vi "Open Controller matrix.vi"(1 "file path (dialog if empty)":path) -> (0 "Cluster":T1)   [LabVIEW 2018]
uses:
  controls/Controller.ctl
  Real-Time/Control Algorithm/Control Algorithm Selection.ctl
  <vilib>/Utility/file.llb/Read Delimited Spreadsheet (DBL).vi
panel:
  out "all rows":dbl[][](array[numeric]) format="%#_24g"
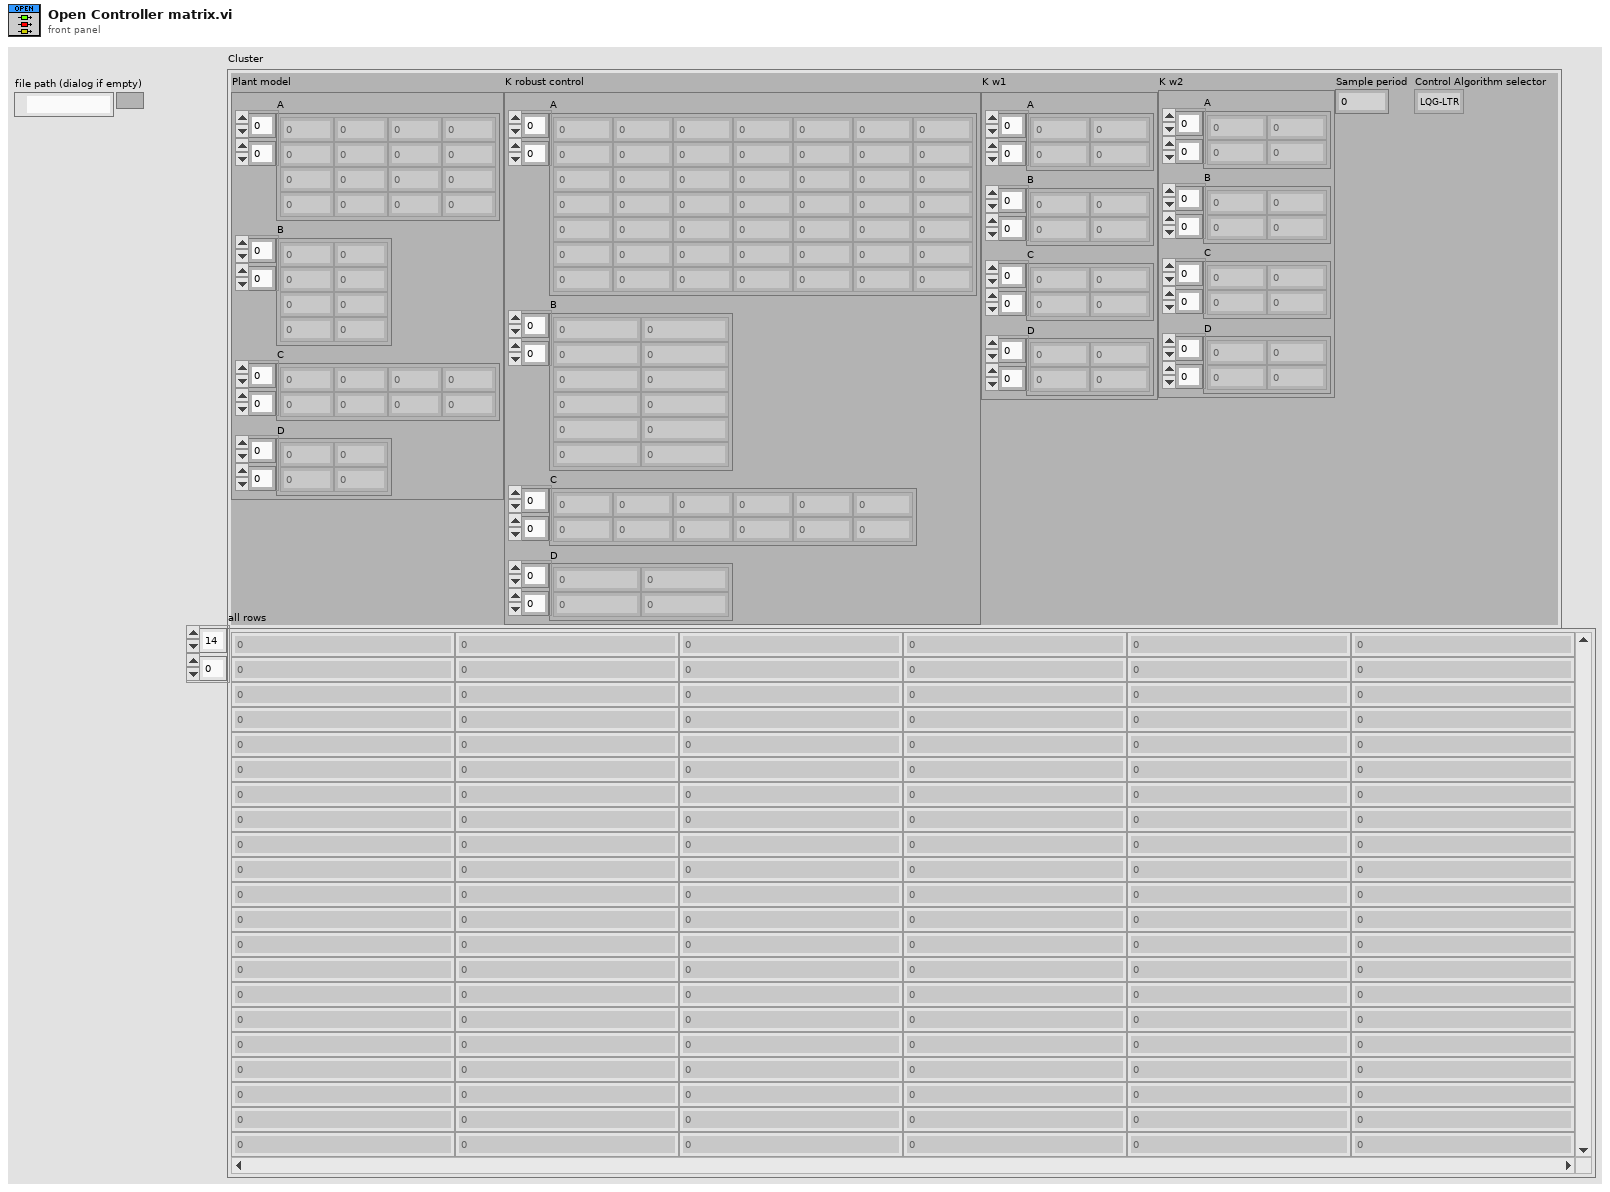
[diagram p1: front panel]
types:
  T1 = typedef "Controller.ctl" = cluster{"Plant model":cluster{"A":dbl[][], "B":dbl[][], "C":dbl[][], "D":dbl[][]}, "K robust control":cluster{"A":dbl[][], "B":dbl[][], "C":dbl[][], "D":dbl[][]}, "K w1":cluster{"A":dbl[][], "B":dbl[][], "C":dbl[][], "D":dbl[][]}, "K w2":cluster{"A":dbl[][], "B":dbl[][], "C":dbl[][], "D":dbl[][]}, "Sample period":dbl, "Control Algorithm selector":T2}
  T2 = typedef "Control Algorithm Selection.ctl" = enum16{"LQG-LTR", "Hinf"}
  T3 = cluster{"A":dbl[][], "B":dbl[][], "C":dbl[][], "D":dbl[][]}
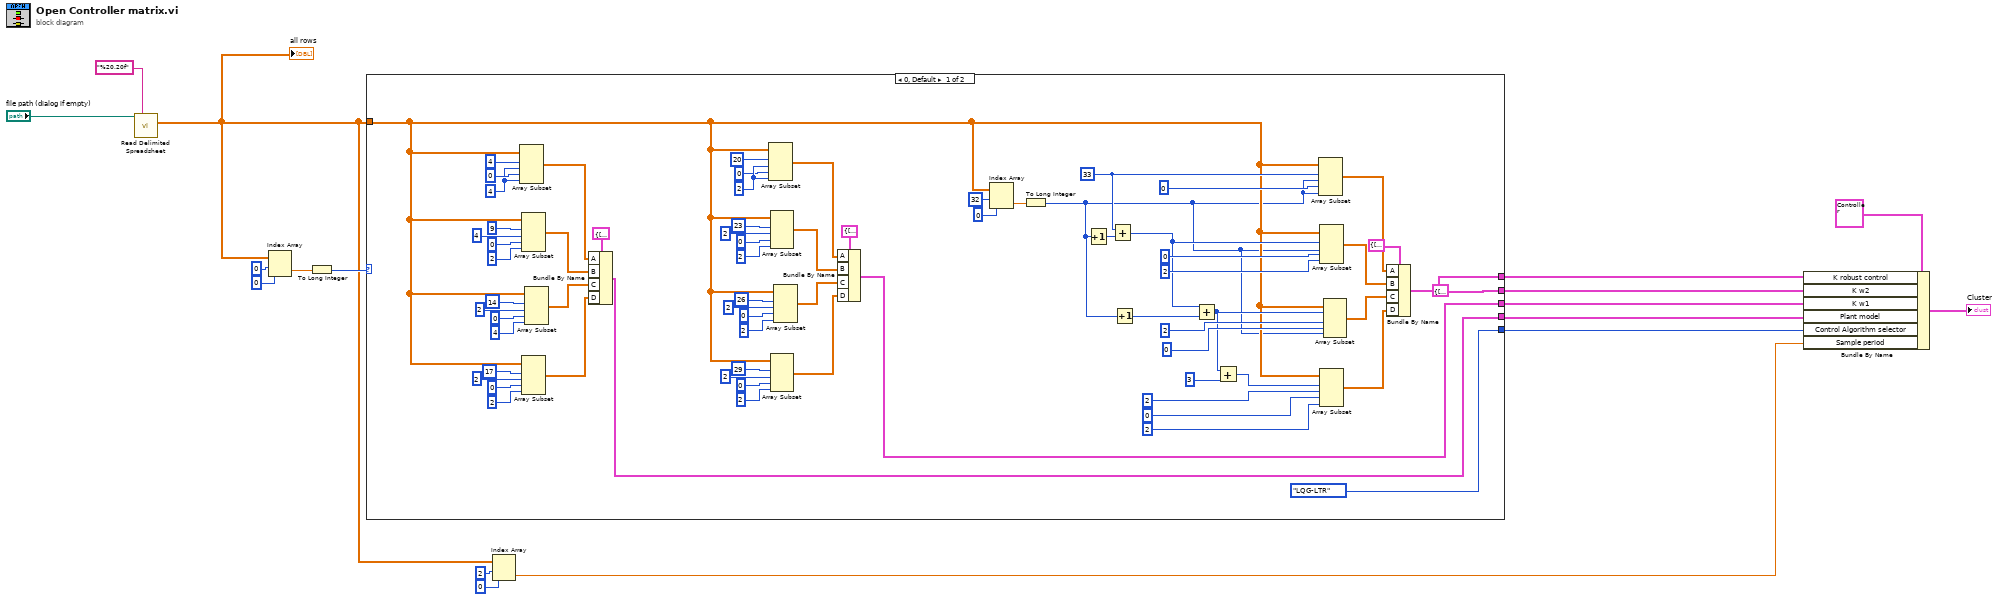
[diagram p0: block diagram]
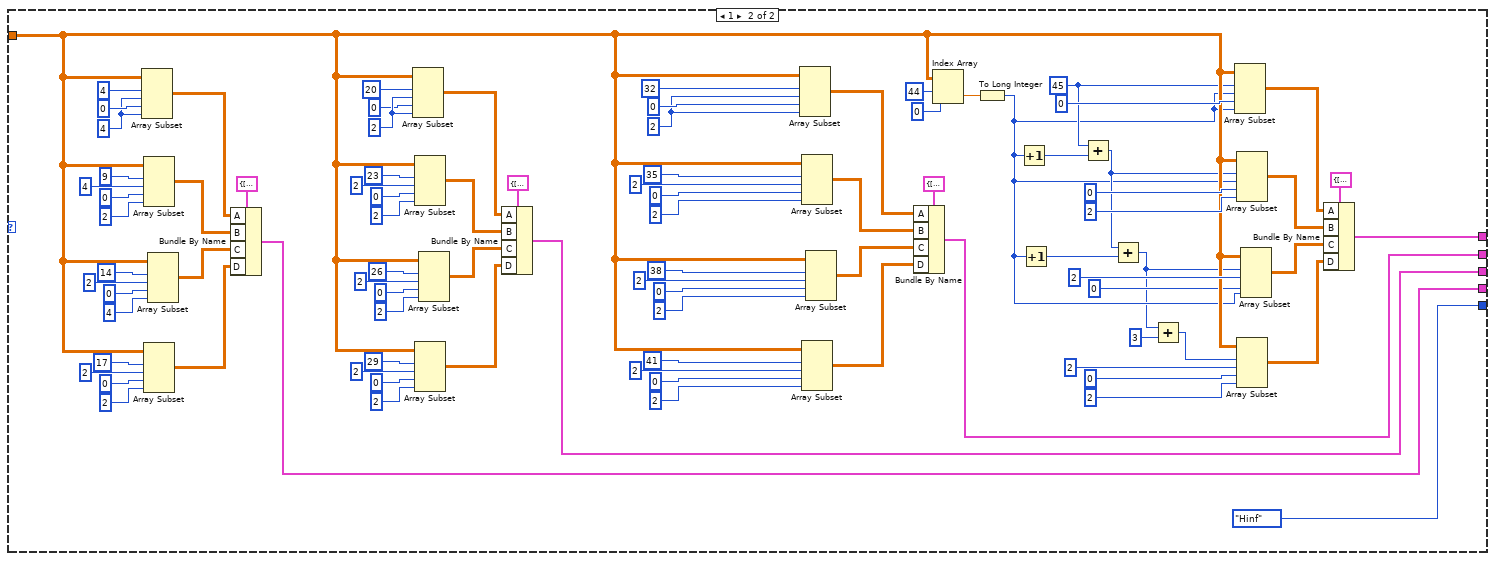
[diagram p2: hidden frame]
diagram:
  n1 = call-poly <vilib>:"Read Delimited Spreadsheet.vi"("file path (dialog if empty)"="file path (dialog if empty)", "format (%.3f)"="%20.20f") -> ("all rows"=w10:dbl[][])  [unwired: 8 in, 5 out]
  "all rows" <- w10
  n2 = Index Array(array=w10, index (row)=0, index (col)=0 ("disabled index (col)")) -> (element=w12:dbl)
  n3 = To Long Integer(number=w12) -> (32bit integer=w11:i32)
  n4 = case shown="0, Default" w11 {
    tunnel: w10 -> [w25 w97]
    tunnel: [T3 {"A"=[], "B"=[], "C"=[], "D"=[]} ("Plant model") w102] -> w9
    tunnel: [w34 w117] -> w8
    tunnel: [w33 w116] -> w7
    tunnel: [Control_Algorithm_Selection."LQG-LTR" ("Control Algorithm selector") Control_Algorithm_Selection."Hinf" ("Control Algorithm selector")] -> w5
    tunnel: [w19 w101] -> w2
    frame 0, Default {
      w31 = 33 ("index")
      w53 = 2 ("index")
      w82 = 4 ("index")
      n5 = Array Subset(array=w25, index (row)=4 ("index"), length (row)=w82, index (col)=0 ("index"), length (col)=w82) -> (w71:dbl[][])
      n6 = Array Subset(array=w25, index (row)=9 ("index"), length (row)=4 ("index"), index (col)=0 ("index"), length (col)=2 ("length")) -> (w70:dbl[][])
      n7 = Array Subset(array=w25, index (row)=17 ("index"), length (row)=2 ("index"), index (col)=0 ("index"), length (col)=2 ("length")) -> (w68:dbl[][])
      n8 = Array Subset(array=w25, index (row)=14 ("index"), length (row)=2 ("index"), index (col)=0 ("index"), length (col)=4 ("length")) -> (w69:dbl[][])
      n9 = Bundle By Name(cluster=T3 {"A"=[[0.998469, 0.0, 0.00419648, 0.0], [0.0, 0.998469, 0.0, 0.00419648], [0.0, 0.0, 0.9958, 0.0], [0.0, 0.0, 0.0, 0.9958]], "B"=[[0.00424088, 5.94248e-06], [5.94248e-06, 0.00424088], [0.0, 0.00282348], [0.00282348, 0.0]], "C"=[[1.0, 0.0, 0.0, 0.0], [0.0, 1.0, 0.0, 0.0]], "D"=[[0.0, 0.0], [0.0, 0.0]]} ("Plant model"), "A"=w71, "B"=w70, "C"=w69, "D"=w68) -> (w33:T3)
      n10 = Array Subset(array=w25, index (row)=20 ("index"), length (row)=w53, index (col)=0 ("index"), length (col)=w53) -> (w64:dbl[][])
      n11 = Array Subset(array=w25, index (row)=23 ("index"), length (row)=2 ("index"), index (col)=0 ("index"), length (col)=2 ("length")) -> (w65:dbl[][])
      n12 = Array Subset(array=w25, index (row)=29 ("index"), length (row)=2 ("index"), index (col)=0 ("index"), length (col)=2 ("length")) -> (w67:dbl[][])
      n13 = Array Subset(array=w25, index (row)=26 ("index"), length (row)=2 ("index"), index (col)=0 ("index"), length (col)=2 ("length")) -> (w66:dbl[][])
      n14 = Bundle By Name(cluster=T3 {"A"=[[0.998469, 0.0, 0.00419648, 0.0], [0.0, 0.998469, 0.0, 0.00419648], [0.0, 0.0, 0.9958, 0.0], [0.0, 0.0, 0.0, 0.9958]], "B"=[[0.00424088, 5.94248e-06], [5.94248e-06, 0.00424088], [0.0, 0.00282348], [0.00282348, 0.0]], "C"=[[1.0, 0.0, 0.0, 0.0], [0.0, 1.0, 0.0, 0.0]], "D"=[[0.0, 0.0], [0.0, 0.0]]} ("Plant model"), "A"=w64, "B"=w65, "C"=w66, "D"=w67) -> (w34:T3)
      n15 = Index Array(array=w25, index (row)=32, index (col)=0 ("disabled index (col)")) -> (element=w22:dbl)
      n16 = To Long Integer(number=w22) -> (32bit integer=w21:i32)
      n17 = Increment(x=w21) -> (x+1=w30:i32)
      n18 = Add(x=w31, y=w30) -> (x+y=w28:i32)
      n19 = Increment(x=w21) -> (x+1=w29:i32)
      n20 = Add(x=w28, y=w29) -> (x+y=w27:i32)
      n21 = Add(x=w27, y=3 ("index")) -> (x+y=w26:i32)
      n22 = Array Subset(array=w25, index (row)=w31, length (row)=w21, index (col)=0 ("index"), length (col)=w21) -> (w38:dbl[][])
      n23 = Array Subset(array=w25, index (row)=w28, length (row)=w21, index (col)=0 ("index"), length (col)=2 ("length")) -> (w37:dbl[][])
      n24 = Array Subset(array=w25, index (row)=w26, length (row)=2 ("index"), index (col)=0 ("index"), length (col)=2 ("length")) -> (w35:dbl[][])
      n25 = Array Subset(array=w25, index (row)=w27, length (row)=2 ("index"), index (col)=0 ("index"), length (col)=w21) -> (w36:dbl[][])
      n26 = Bundle By Name(cluster=T3 {"A"=[[0.998469, 0.0, 0.00419648, 0.0], [0.0, 0.998469, 0.0, 0.00419648], [0.0, 0.0, 0.9958, 0.0], [0.0, 0.0, 0.0, 0.9958]], "B"=[[0.00424088, 5.94248e-06], [5.94248e-06, 0.00424088], [0.0, 0.00282348], [0.00282348, 0.0]], "C"=[[1.0, 0.0, 0.0, 0.0], [0.0, 1.0, 0.0, 0.0]], "D"=[[0.0, 0.0], [0.0, 0.0]]} ("Plant model"), "A"=w38, "B"=w37, "C"=w36, "D"=w35) -> (w19:T3)
    }
    frame 1 {
      w95 = 45 ("index")
      w132 = 2 ("index")
      w143 = 2 ("index")
      w172 = 4 ("index")
      n27 = Array Subset(array=w97, index (row)=4 ("index"), length (row)=w172, index (col)=0 ("index"), length (col)=w172) -> (w161:dbl[][])
      n28 = Array Subset(array=w97, index (row)=9 ("index"), length (row)=4 ("index"), index (col)=0 ("index"), length (col)=2 ("length")) -> (w160:dbl[][])
      n29 = Array Subset(array=w97, index (row)=17 ("index"), length (row)=2 ("index"), index (col)=0 ("index"), length (col)=2 ("length")) -> (w158:dbl[][])
      n30 = Array Subset(array=w97, index (row)=14 ("index"), length (row)=2 ("index"), index (col)=0 ("index"), length (col)=4 ("length")) -> (w159:dbl[][])
      n31 = Bundle By Name(cluster=T3 {"A"=[[0.998469, 0.0, 0.00419648, 0.0], [0.0, 0.998469, 0.0, 0.00419648], [0.0, 0.0, 0.9958, 0.0], [0.0, 0.0, 0.0, 0.9958]], "B"=[[0.00424088, 5.94248e-06], [5.94248e-06, 0.00424088], [0.0, 0.00282348], [0.00282348, 0.0]], "C"=[[1.0, 0.0, 0.0, 0.0], [0.0, 1.0, 0.0, 0.0]], "D"=[[0.0, 0.0], [0.0, 0.0]]} ("Plant model"), "A"=w161, "B"=w160, "C"=w159, "D"=w158) -> (w116:T3)
      n32 = Array Subset(array=w97, index (row)=20 ("index"), length (row)=w143, index (col)=0 ("index"), length (col)=w143) -> (w154:dbl[][])
      n33 = Array Subset(array=w97, index (row)=23 ("index"), length (row)=2 ("index"), index (col)=0 ("index"), length (col)=2 ("length")) -> (w155:dbl[][])
      n34 = Array Subset(array=w97, index (row)=29 ("index"), length (row)=2 ("index"), index (col)=0 ("index"), length (col)=2 ("length")) -> (w157:dbl[][])
      n35 = Array Subset(array=w97, index (row)=26 ("index"), length (row)=2 ("index"), index (col)=0 ("index"), length (col)=2 ("length")) -> (w156:dbl[][])
      n36 = Bundle By Name(cluster=T3 {"A"=[[0.998469, 0.0, 0.00419648, 0.0], [0.0, 0.998469, 0.0, 0.00419648], [0.0, 0.0, 0.9958, 0.0], [0.0, 0.0, 0.0, 0.9958]], "B"=[[0.00424088, 5.94248e-06], [5.94248e-06, 0.00424088], [0.0, 0.00282348], [0.00282348, 0.0]], "C"=[[1.0, 0.0, 0.0, 0.0], [0.0, 1.0, 0.0, 0.0]], "D"=[[0.0, 0.0], [0.0, 0.0]]} ("Plant model"), "A"=w154, "B"=w155, "C"=w156, "D"=w157) -> (w117:T3)
      n37 = Array Subset(array=w97, index (row)=32 ("index"), length (row)=w132, index (col)=0 ("index"), length (col)=w132) -> (w121:dbl[][])
      n38 = Array Subset(array=w97, index (row)=35 ("index"), length (row)=2 ("index"), index (col)=0 ("index"), length (col)=2 ("length")) -> (w120:dbl[][])
      n39 = Array Subset(array=w97, index (row)=41 ("index"), length (row)=2 ("index"), index (col)=0 ("index"), length (col)=2 ("length")) -> (w118:dbl[][])
      n40 = Array Subset(array=w97, index (row)=38 ("index"), length (row)=2 ("index"), index (col)=0 ("index"), length (col)=2 ("length")) -> (w119:dbl[][])
      n41 = Bundle By Name(cluster=T3 {"A"=[[0.998469, 0.0, 0.00419648, 0.0], [0.0, 0.998469, 0.0, 0.00419648], [0.0, 0.0, 0.9958, 0.0], [0.0, 0.0, 0.0, 0.9958]], "B"=[[0.00424088, 5.94248e-06], [5.94248e-06, 0.00424088], [0.0, 0.00282348], [0.00282348, 0.0]], "C"=[[1.0, 0.0, 0.0, 0.0], [0.0, 1.0, 0.0, 0.0]], "D"=[[0.0, 0.0], [0.0, 0.0]]} ("Plant model"), "A"=w121, "B"=w120, "C"=w119, "D"=w118) -> (w102:T3)
      n42 = Index Array(array=w97, index (row)=44, index (col)=0 ("disabled index (col)")) -> (element=w98:dbl)
      n43 = To Long Integer(number=w98) -> (32bit integer=w92:i32)
      n44 = Increment(x=w92) -> (x+1=w96:i32)
      n45 = Increment(x=w92) -> (x+1=w91:i32)
      n46 = Add(x=w95, y=w96) -> (x+y=w93:i32)
      n47 = Add(x=w93, y=w91) -> (x+y=w90:i32)
      n48 = Add(x=w90, y=3) -> (x+y=w88:i32)
      n49 = Array Subset(array=w97, index (row)=w95, length (row)=w92, index (col)=0 ("index"), length (col)=w92) -> (w106:dbl[][])
      n50 = Array Subset(array=w97, index (row)=w93, length (row)=w92, index (col)=0 ("index"), length (col)=2 ("length")) -> (w105:dbl[][])
      n51 = Array Subset(array=w97, index (row)=w88, length (row)=2 ("index"), index (col)=0 ("index"), length (col)=2 ("length")) -> (w103:dbl[][])
      n52 = Array Subset(array=w97, index (row)=w90, length (row)=2 ("index"), index (col)=0 ("index"), length (col)=w92) -> (w104:dbl[][])
      n53 = Bundle By Name(cluster=T3 {"A"=[[0.998469, 0.0, 0.00419648, 0.0], [0.0, 0.998469, 0.0, 0.00419648], [0.0, 0.0, 0.9958, 0.0], [0.0, 0.0, 0.0, 0.9958]], "B"=[[0.00424088, 5.94248e-06], [5.94248e-06, 0.00424088], [0.0, 0.00282348], [0.00282348, 0.0]], "C"=[[1.0, 0.0, 0.0, 0.0], [0.0, 1.0, 0.0, 0.0]], "D"=[[0.0, 0.0], [0.0, 0.0]]} ("Plant model"), "A"=w106, "B"=w105, "C"=w104, "D"=w103) -> (w101:T3)
    }
  }
  n54 = Index Array(array=w10, index (row)=2, index (col)=0 ("disabled index (col)")) -> (element=w6:dbl)
  n55 = Bundle By Name(cluster=T1 {"Plant model"={"A"=[], "B"=[], "C"=[], "D"=[]}, "K robust control"={"A"=[], "B"=[], "C"=[], "D"=[]}, "K w1"={"A"=[], "B"=[], "C"=[], "D"=[]}, "K w2"={"A"=[], "B"=[], "C"=[], "D"=[]}, "Sample period"=0.0, "Control Algorithm selector"=enum."LQG-LTR"} ("Cluster"), "K robust control"=w2, "K w2"=w9, "K w1"=w8, "Plant model"=w7, "Control Algorithm selector"=w5, "Sample period"=w6) -> (→"Cluster":T1)
